vi "Teleop.vi"(1 "PreValue 2":bool, 3 "PreValue":bool, 10 "Match Info":T1={"Autonomous Elapsed Seconds"=0.0, "TeleOp Elapsed Seconds"=0.0, "Disabled Elapsed Seconds"=0.0, "Visited Autonomous"=FALSE, "Visited TeleOp"=FALSE, "Visited Disabled"=FALSE, "Autonomous Settings"={"Autonomous Style"=enum."Independent", "VI Refnum"=refnum}}, 11 "Call Context":T2) -> (0 "CurrentValue 2":bool, 2 "CurrentValue":bool)   [LabVIEW 2015]
doc: "This VI is called for each TeleOp packet received from the DS where the robot is not disabled. It is often used to read from the joysticks and update I/O or to update setpoints for timed control loops. It should complete and return within 20 milliseconds or it may miss DS packets."
uses:
  <vilib>/Rock Robotics/WPI/DriverStation/WPI_DriverStationDerivedRobotMode.ctl
  <vilib>/Rock Robotics/WPI/DriverStation/WPI_DriverStationMatch Info.ctl
  <vilib>/Rock Robotics/WPI/Solenoid/WPI_SolenoidValue.ctl
  <vilib>/Rock Robotics/WPI/Utilities/WPI_GetSetVariantRefNum.vi
  <vilib>/Rock Robotics/Network Tables/NT Write Boolean.vi
  <vilib>/Rock Robotics/Network Tables/NT Write Numeric Array.vi
  <vilib>/Rock Robotics/Network Tables/NT Read Boolean.vi
  <vilib>/Rock Robotics/Network Tables/NT Read Number.vi
  <vilib>/Rock Robotics/WPI/Solenoid/WPI_SolenoidSetEnum.vi
panel:
  out "Sample Slider 0":dbl(slide) scale=0.0..5.0
  out "Sample Boolean 1":bool
  out "Sample Boolean 0":bool
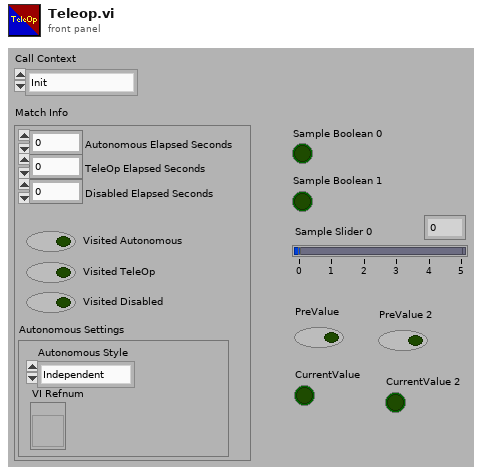
[diagram p1: front panel]
types:
  T1 = typedef "WPI_DriverStationMatch Info.ctl" = cluster{"Autonomous Elapsed Seconds":dbl, "TeleOp Elapsed Seconds":dbl, "Disabled Elapsed Seconds":dbl, "Visited Autonomous":bool, "Visited TeleOp":bool, "Visited Disabled":bool, "Autonomous Settings":cluster{"Autonomous Style":enum16{"Iterative", "Independent"}, "VI Refnum":refnum<vi>}}
  T2 = typedef "WPI_DriverStationDerivedRobotMode.ctl" = enum16{"Init", "Execute", "Stop"}
  T3 = typedef "WPI_SolenoidValue.ctl" = enum16{"Off", "On", "Forward", "Reverse"}
  T4 = typedef "WPI_RobotDriveDevRef.ctl" = cluster{"DevStatus":errorcluster, "Motors[]":T5[], "Square Inputs":bool, "Max Output":dbl}
  T5 = typedef "WPI_MotorControlDeviceRef.ctl" = cluster{"DeviceStatus":errorcluster, "Type":T6, "PWM":cluster{"PWM Channel":T7, "DeadBand":T8}, "CAN":cluster{"Device Number":u8, "Control Mode":T9, "Semaphore":T10, "Max Vout":dbl, "TalonSRX Control Mode":T11}, "Invert":bool}
  T6 = typedef "WPI_MotorControlType.ctl" = enum16{"PWM", "CAN", "CANTalonSRX"}
  T7 = typedef "FPGA_DIOPWMChannel.ctl" = enum8{"PWM 0", "PWM 1", "PWM 2", "PWM 3", "PWM 4", "PWM 5", "PWM 6", "PWM 7", "PWM 8", "PWM 9", "PWM MXP 0", "PWM MXP 1", "PWM MXP 2", "PWM MXP 3", "PWM MXP 4", "PWM MXP 5", "PWM MXP 6", "PWM MXP 7", "PWM MXP 8", "PWM MXP 9", "Invalid"}
  T8 = typedef "WPI_PWMDeadband.ctl" = cluster{"Name":string, "maxPositivePwm":i32, "minPositivePwm":i32, "centerPwm":i32, "maxNegativePwm":i32, "minNegativePwm":i32, "angularRange":u16}
  T9 = typedef "WPI_CANJaguar_ControlMode.ctl" = enum8{"Percent VBus", "Current", "Speed", "Position", "Voltage"}
  T10 = typedef "Semaphore RefNum" = refnum<k1>
  T11 = typedef "WPI_CANTalonSRX_APIControlMode.ctl" = enum8{"Percent VBus", "Speed", "Position", "Slave", "Unchanged / Invalid", "Voltage Compensation", "Current", "Motion Profile"}
  T12 = typedef "WPI_JoystickDevRef.ctl" = cluster{"Device":T13}
  T13 = typedef "WPI_JoystickDeviceEnum.ctl" = enum16{"USB 0", "USB 1", "USB 2", "USB 3", "USB 4", "USB 5"}
  T14 = cluster{"Buttons[0]":bool, "Buttons[1]":bool, "Buttons[2]":bool, "Buttons[3]":bool, "Buttons[4]":bool, "Buttons[5]":bool, "Buttons[6]":bool, "Buttons[7]":bool, "Buttons[8]":bool}
  T15 = typedef "WPI_DigitalInputDevRef.ctl" = cluster{"DevStatus":errorcluster, "DIO Channel":T16}
  T16 = typedef "FPGA_DIOChannel.ctl" = enum8{"DIO 0", "DIO 1", "DIO 2", "DIO 3", "DIO 4", "DIO 5", "DIO 6", "DIO 7", "DIO 8", "DIO 9", "DIO MXP 0", "DIO MXP 1", "DIO MXP 2", "DIO MXP 3", "DIO MXP 4", "DIO MXP 5", "DIO MXP 6", "DIO MXP 7", "DIO MXP 8", "DIO MXP 9", "DIO MXP 10", "DIO MXP 11", "DIO MXP 12", "DIO MXP 13", "DIO MXP 14", "DIO MXP 15", "Invalid"}
  T17 = typedef "WPI_SolenoidDevRef.ctl" = cluster{"DevStatus":errorcluster, "Pneumatics Control Module":u8, "Forward Solenoid Channel":T18, "Reverse Solenoid Channel":T18}
  T18 = typedef "WPI_SolenoidChannel.ctl" = enum8{"Solenoid 0", "Solenoid 1", "Solenoid 2", "Solenoid 3", "Solenoid 4", "Solenoid 5", "Solenoid 6", "Solenoid 7", "Invalid"}
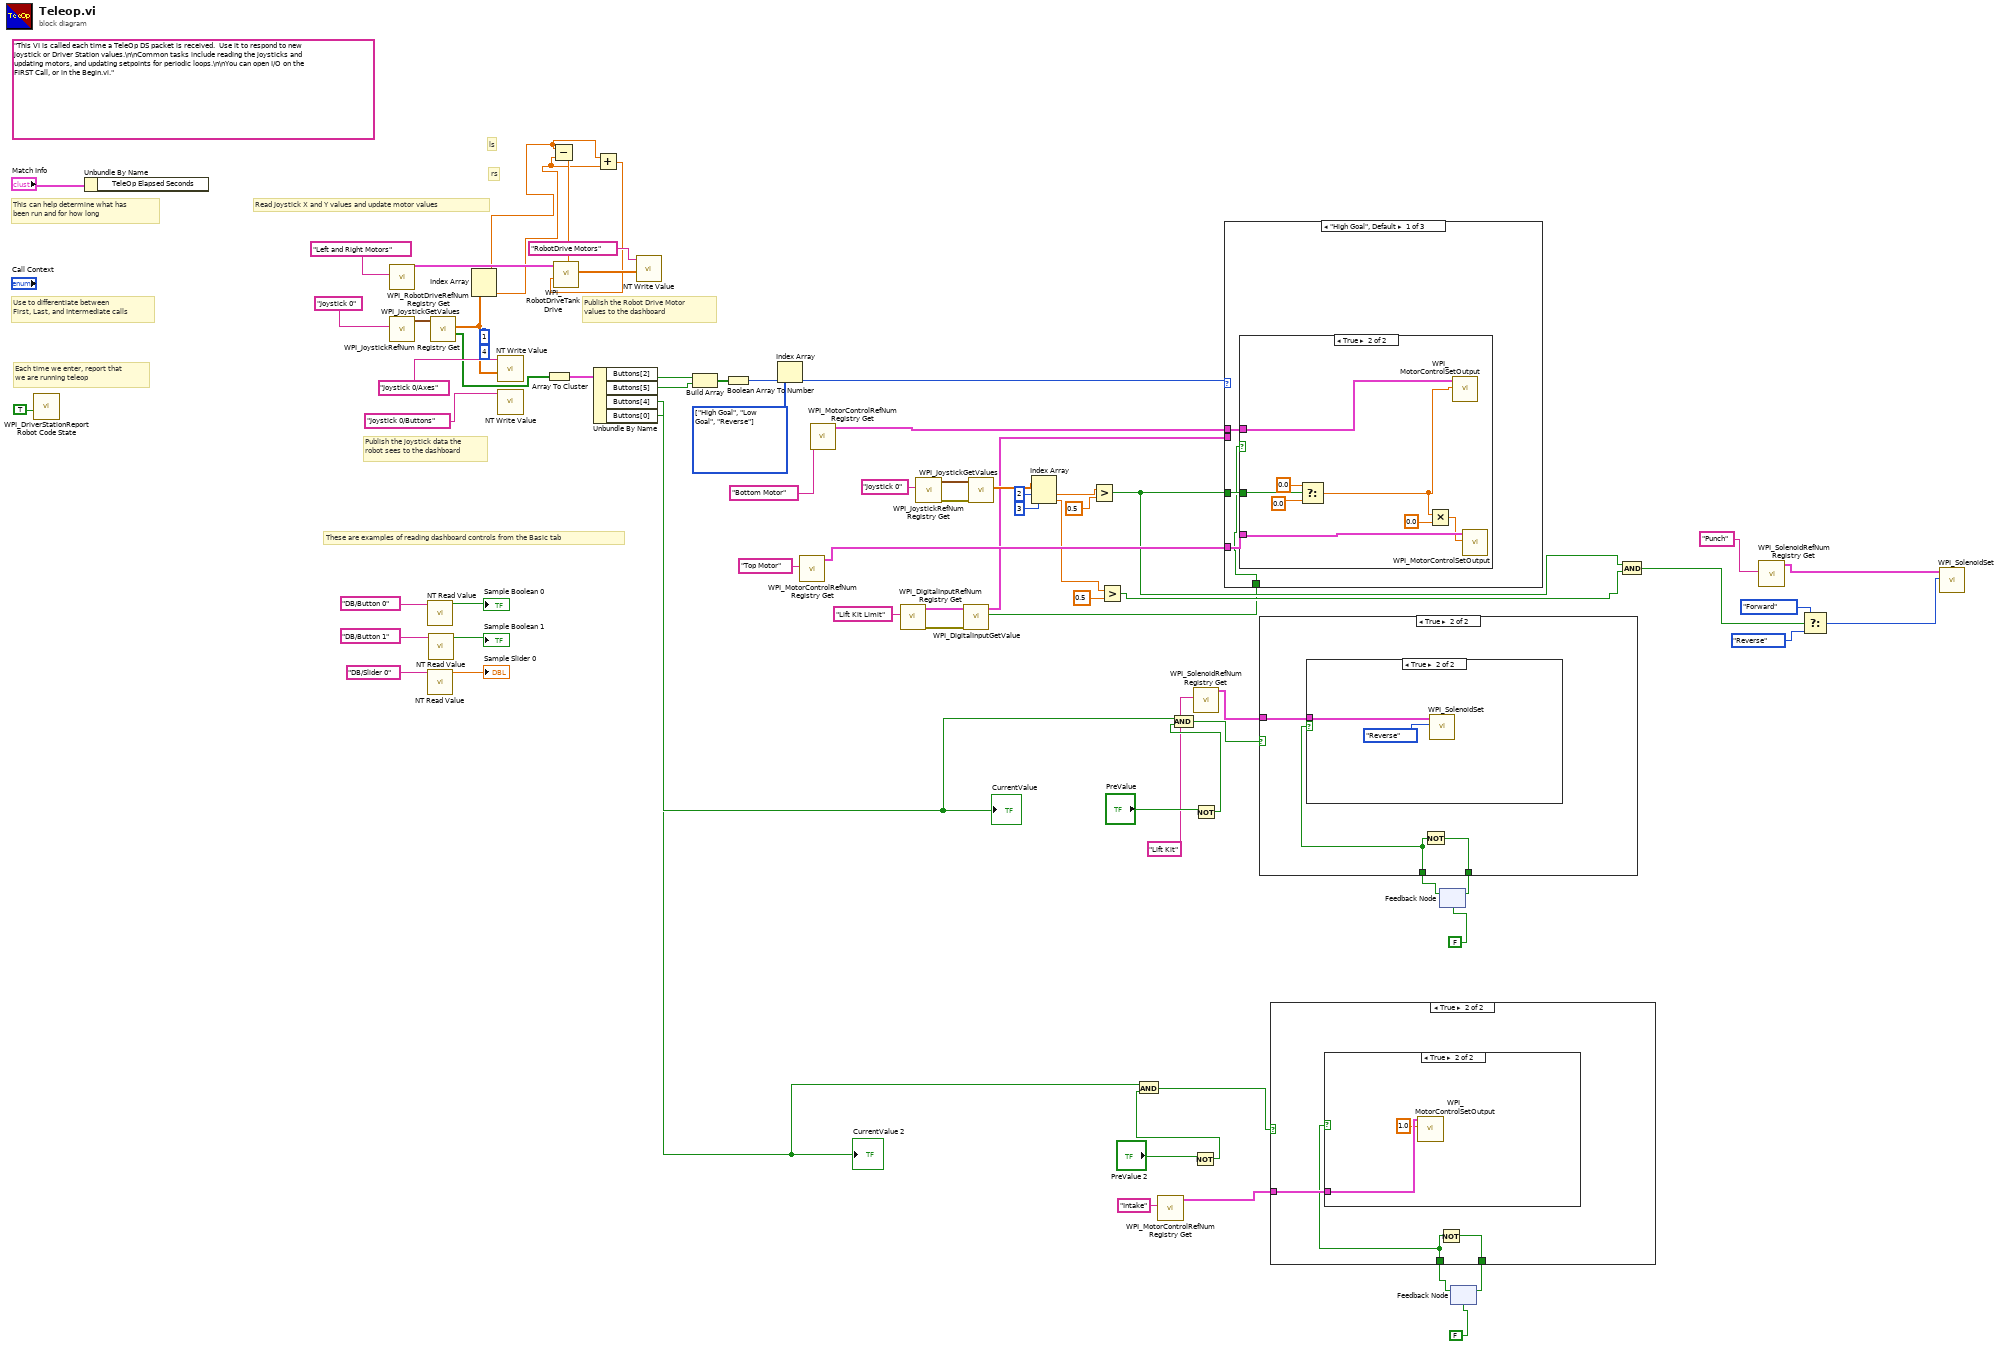
[diagram p0: block diagram]
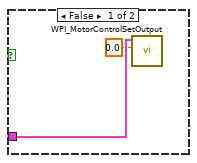
[diagram p3: hidden frame]
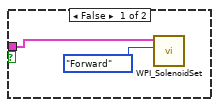
[diagram p5: hidden frame]
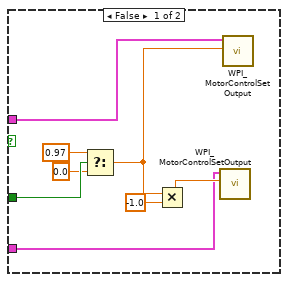
[diagram p6: hidden frame]
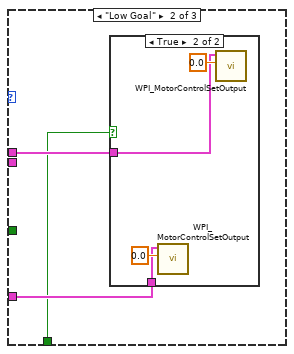
[diagram p7: hidden frame]
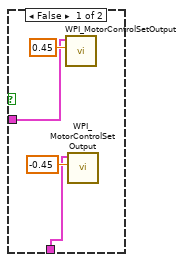
[diagram p8: hidden frame]
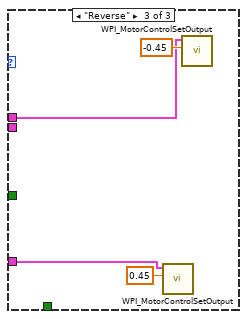
[diagram p9: hidden frame]
diagram:
  w57 = enum16{"High Goal", "Low Goal", "Reverse", ""}[] [enum."High Goal", enum."Low Goal", enum."Reverse"] items=["High Goal", "Low Goal", "Reverse", ""] ("array")
  (unwired) "This VI is called each time a TeleOp DS packet is received.  Use it to respond to new joystick or Driver Station values.\n\nCommon tasks include reading the joysticks and updating motors, and updating setpoints for periodic loops.\n\nYou can open I/O on the FIRST Call, or in the Begin.vi."
  # "rs"
  # "ls"
  # "These are examples of reading dashboard controls from the Basic tab"
  # "Publish the Robot Drive Motor\nvalues to the dashboard"
  # "Publish the joystick data the\nrobot sees to the dashboard"
  # "Each time we enter, report that\nwe are running teleop"
  # "Use to differentiate between\nFirst, Last, and Intermediate calls"
  # "This can help determine what has\nbeen run and for how long"
  # "Read Joystick X and Y values and update motor values"
  n1 = call <vilib>:"WPI_DriverStationReport Robot Code State.vi"("TeleOp"=TRUE ("Autonomous")) -> ()  [unwired: 10 in, 1 out]
  n2 = Unbundle By Name("Match Info") -> ()  [unwired: 1 out]
  n3 = call <vilib>:"WPI_RobotDriveRefNum Registry Get.vi"("refnum name"="Left and Right Motors") -> ("RobotDriveDevRef"=w40:T4)  [unwired: 1 in, 9 out]
  n4 = call <vilib>:"WPI_JoystickRefNum Registry Get.vi"("refnum name"="Joystick 0") -> ("JoystickDevRef"=w73:T12)  [unwired: 1 in, 9 out]
  n5 = call-poly <vilib>:"NT Read Value.vi"("Name"="DB/Button 0" ("refnum name")) -> ("Boolean"=→"Sample Boolean 0":bool)  [unwired: 9 in, 1 out]
  n6 = call-poly <vilib>:"NT Read Value.vi"("Name"="DB/Slider 0" ("refnum name")) -> ("Numeric"=→"Sample Slider 0":dbl)  [unwired: 9 in, 1 out]
  n7 = call-poly <vilib>:"NT Read Value.vi"("Name"="DB/Button 1" ("refnum name")) -> ("Boolean"=→"Sample Boolean 1":bool)  [unwired: 9 in, 1 out]
  n8 = call <vilib>:"WPI_JoystickGetValues.vi"("JoystickDevRef"=w73) -> ("Buttons"=w53:bool[], "Axes"=w69:dbl[])  [unwired: 6 in, 3 out]
  n9 = Index Array(array=w69, index #1=1 ("index"), index #2=4 ("index")) -> (element #1=w37:dbl, element #2=w36:dbl)
  n10 = call-poly <vilib>:"NT Write Value.vi"("Numeric Array"=w69, "Name"="Joystick 0/Axes") -> ()  [unwired: 9 in, 1 out]
  n11 = call-poly <vilib>:"NT Write Value.vi"("Name"="Joystick 0/Buttons") -> ()  [unwired: 10 in, 1 out]
  n12 = Array To Cluster(array=w53) -> (cluster=w61:T14)
  n13 = Subtract(x=w37, y=w36) -> (x-y=w38:dbl)
  n14 = Unbundle By Name(w61) -> ("Buttons[2]"=w33:bool, "Buttons[5]"=w60:bool, "Buttons[4]"=w50:bool, "Buttons[0]"=w8:bool)
  "CurrentValue" <- w50
  "CurrentValue 2" <- w8
  n15 = Add(x=w37, y=w36) -> (x+y=w39:dbl)
  n16 = call <vilib>:"WPI_RobotDriveTankDrive.vi"("Right axis value"=w39, "Left axis value"=w38, "RobotDriveDevRef"=w40) -> ("Motor Values"=w41:dbl[])  [unwired: 6 in, 2 out]
  n17 = call-poly <vilib>:"NT Write Value.vi"("Numeric Array"=w41, "Name"="RobotDrive Motors") -> ()  [unwired: 9 in, 1 out]
  n18 = Build Array(w33, w60) -> (w59:bool[])
  n19 = Boolean Array To Number(Boolean array=w59) -> (number=w58:u32)
  n20 = Index Array(array=w57, index=w58) -> (element=w56:enum16{"High Goal", "Low Goal", "Reverse", ""})
  n21 = call <vilib>:"WPI_MotorControlRefNum Registry Get.vi"("refnum name"="Top Motor") -> ("MotorControlDevRef"=w51:T5)  [unwired: 9 in, 1 out]
  n22 = call <vilib>:"WPI_MotorControlRefNum Registry Get.vi"("refnum name"="Bottom Motor") -> ("MotorControlDevRef"=w55:T5)  [unwired: 9 in, 1 out]
  n23 = call <vilib>:"WPI_DigitalInputRefNum Registry Get.vi"("refnum name"="Lift Kit Limit") -> ("error out"=w3:errorcluster, "DigitalInputDevRef"=w5:T15)  [unwired: 9 in]
  n24 = call <vilib>:"WPI_JoystickRefNum Registry Get.vi"("refnum name"="Joystick 0") -> ("error out"=w31:errorcluster, "JoystickDevRef"=w30:T12)  [unwired: 1 in, 8 out]
  n25 = call <vilib>:"WPI_DigitalInputGetValue.vi"("error in (no error)"=w3, "DigitalInputDevRef"=w5) -> ("Value"=w1:bool, "DigitalInputDevRef"=w2:T15)  [unwired: 7 in, 1 out]
  n26 = call <vilib>:"WPI_JoystickGetValues.vi"("error in (no error)"=w31, "JoystickDevRef"=w30) -> ("Axes"=w28:dbl[])  [unwired: 5 in, 4 out]
  n27 = Index Array(array=w28, index #1=2 ("index"), index #2=3 ("index")) -> (element #1=w27:dbl, element #2=w22:dbl)
  n28 = Greater?(x=w27, y=0.5) -> (0:w25:bool)
  n29 = Greater?(x=w22, y=0.5) -> (0:w21:bool)
  n30 = call <vilib>:"WPI_MotorControlRefNum Registry Get.vi"("refnum name"="Intake") -> ("MotorControlDevRef"=w10:T5)  [unwired: 9 in, 1 out]
  n31 = Not(x="PreValue 2") -> (.not. x?=w7:bool)
  n32 = And(x=w8, y=w7) -> (x .and. y?=w6:bool)
  n33 = call <vilib>:"WPI_SolenoidRefNum Registry Get.vi"("refnum name"="Lift Kit") -> ("SolenoidDevRef"=w42:T17)  [unwired: 9 in, 1 out]
  n34 = Not(x="PreValue") -> (.not. x?=w48:bool)
  n35 = And(x=w50, y=w48) -> (x .and. y?=w47:bool)
  n36 = case shown="\"High Goal\", Default" w56 {
    tunnel: w55 -> [w80 w99 w110]
    tunnel: w51 -> [w79 w98 w108]
    tunnel: w25 -> [w78 _ _]
    tunnel: w2 -> [_ _ _]
    tunnel: w1 -> [w77 w97 _]
    frame "High Goal", Default {
      n37 = case shown="True" w77 {
        tunnel: w80 -> [w82 w96]
        tunnel: w79 -> [w81 w95]
        tunnel: w78 -> [w87 w94]
        frame False {
          n38 = Select(t=0.97, s=w87, f=0.0) -> (s? t:f=w86:dbl)
          n39 = Multiply(x=w86, y=-1.0) -> (x*y=w88:dbl)
          n40 = call <vilib>:"WPI_MotorControlSetOutput.vi"("Output"=w88, "MotorControlDevRef"=w81) -> ()  [unwired: 7 in, 3 out]
          n41 = call <vilib>:"WPI_MotorControlSetOutput.vi"("Output"=w86, "MotorControlDevRef"=w82) -> ()  [unwired: 7 in, 3 out]
        }
        frame True {
          n42 = Select(t=0.0, s=w94, f=0.0) -> (s? t:f=w92:dbl)
          n43 = Multiply(x=w92, y=0.0) -> (x*y=w90:dbl)
          n44 = call <vilib>:"WPI_MotorControlSetOutput.vi"("Output"=w92, "MotorControlDevRef"=w96) -> ()  [unwired: 7 in, 3 out]
          n45 = call <vilib>:"WPI_MotorControlSetOutput.vi"("Output"=w90, "MotorControlDevRef"=w95) -> ()  [unwired: 7 in, 3 out]
        }
      }
    }
    frame "Low Goal" {
      n46 = case shown="True" w97 {
        tunnel: w99 -> [w100 w106]
        tunnel: w98 -> [w101 w104]
        frame False {
          n47 = call <vilib>:"WPI_MotorControlSetOutput.vi"("Output"=0.45, "MotorControlDevRef"=w100) -> ()  [unwired: 7 in, 3 out]
          n48 = call <vilib>:"WPI_MotorControlSetOutput.vi"("Output"=-0.45, "MotorControlDevRef"=w101) -> ()  [unwired: 7 in, 3 out]
        }
        frame True {
          n49 = call <vilib>:"WPI_MotorControlSetOutput.vi"("Output"=0.0, "MotorControlDevRef"=w104) -> ()  [unwired: 7 in, 3 out]
          n50 = call <vilib>:"WPI_MotorControlSetOutput.vi"("Output"=0.0, "MotorControlDevRef"=w106) -> ()  [unwired: 7 in, 3 out]
        }
      }
    }
    frame "Reverse" {
      n51 = call <vilib>:"WPI_MotorControlSetOutput.vi"("Output"=0.45, "MotorControlDevRef"=w108) -> ()  [unwired: 7 in, 3 out]
      n52 = call <vilib>:"WPI_MotorControlSetOutput.vi"("Output"=-0.45, "MotorControlDevRef"=w110) -> ()  [unwired: 7 in, 3 out]
    }
  }
  n53 = feedback #1(FALSE) -> (w44:bool)
  n54 = case shown="True" w47 {
    tunnel: [w112 w115] -> w45
    tunnel: w44 -> [w112 w113]
    tunnel: w42 -> [_ w114]
    frame False {
    }
    frame True {
      n55 = case shown="True" w113 {
        tunnel: w114 -> [w117 w119]
        frame False {
          n56 = call-poly <vilib>:"WPI_SolenoidSet.vi"("Value"=WPI_SolenoidValue."Forward", "SolenoidDevRef"=w117) -> ()  [unwired: 8 in, 2 out]
        }
        frame True {
          n57 = call-poly <vilib>:"WPI_SolenoidSet.vi"("Value"=WPI_SolenoidValue."Reverse", "SolenoidDevRef"=w119) -> ()  [unwired: 8 in, 2 out]
        }
      }
      n58 = Not(x=w113) -> (.not. x?=w115:bool)
    }
  }
  n59 = feedback-in #1(w45) -> ()
  n60 = feedback #2(FALSE) -> (w11:bool)
  n61 = case shown="True" w6 {
    tunnel: [w120 w123] -> w12
    tunnel: w11 -> [w120 w121]
    tunnel: w10 -> [_ w122]
    frame False {
    }
    frame True {
      n62 = case shown="True" w121 {
        tunnel: w122 -> [w125 w127]
        frame False {
          n63 = call <vilib>:"WPI_MotorControlSetOutput.vi"("Output"=0.0, "MotorControlDevRef"=w125) -> ()  [unwired: 7 in, 3 out]
        }
        frame True {
          n64 = call <vilib>:"WPI_MotorControlSetOutput.vi"("Output"=1.0, "MotorControlDevRef"=w127) -> ()  [unwired: 7 in, 3 out]
        }
      }
      n65 = Not(x=w121) -> (.not. x?=w123:bool)
    }
  }
  n66 = feedback-in #2(w12) -> ()
  n67 = And(x=w25, y=w21) -> (x .and. y?=w19:bool)
  n68 = call <vilib>:"WPI_SolenoidRefNum Registry Get.vi"("refnum name"="Punch") -> ("SolenoidDevRef"=w20:T17)  [unwired: 9 in, 1 out]
  n69 = Select(t=WPI_SolenoidValue."Forward" ("Value"), s=w19, f=WPI_SolenoidValue."Reverse" ("Value")) -> (s? t:f=w18:T3)
  n70 = call-poly <vilib>:"WPI_SolenoidSet.vi"("Value"=w18, "SolenoidDevRef"=w20) -> ()  [unwired: 8 in, 2 out]
